vi "GFGstringGet.vi"(11 "Variable Name in":string) -> (3 "String":string)   [LabVIEW 2012, in "GFG library.lvlib"]
uses:
  GFG library.lvlib
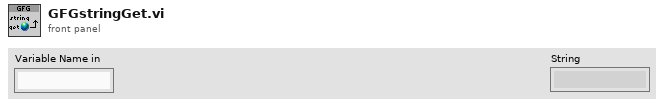
[diagram p1: front panel]
types:
  T1 = typedef "VariantType.lvlib/Type.ctl" = enum8{"Invalid Type", "Void", "I8", "I16", "I32", "I64", "U8", "U16", "U32", "U64", "Single Float", "Double Float", "Extended Float", "Single Complex", "Double Complex", "Extended Complex", "Enum U8", "Enum U16", "Enum U32", "Enum U64", "Single Float With Unit", "Double Float With Unit", "Extended Float With Unit", "Single Complex with Unit", "Double Complex with Unit", "Extended Complex with Unit", "Boolean", "String", "Path", "Picture", "Tag", "Array", "Cluster", "Variant", "LV Variant", "Waveform", "Timestamp", "Digital Waveform", "Digital Data", "ExpressData", "Refnum", "External Data", "VI", "Poly VI", "LabVIEW Class Instance", "Fixed Point"}
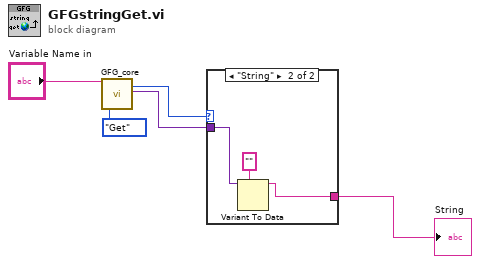
[diagram p0: block diagram]
diagram:
  n1 = call "GFG_core.vi"("Variable Name in"="Variable Name in", "Action"=enum16{"Init", "Set", "Get"}."Get") -> ("Data Type Out"=w4:T1, "Variant Out"=w3:variant)  [unwired: 11 in, 5 out]
  n2 = case shown="\"String\"" w4 {
    tunnel: w3 -> [_ w8]
    tunnel: [_ w6] -> w1
    frame Default {
    }
    frame "String" {
      n3 = Variant To Data(type="" ("Variable Name Out"), Variant=w8) -> (data=w6:string)  [unwired: 1 in, 1 out]
    }
  }
  "String" <- w1
